vi "Get Refs of GUI Objects inside SomeTemplatesFound Tab.vi"(1 "GUI Objects":T1) -> (0 "Refs of GUI Objects inside SomeTemplatesFound Tab":refnum<vi>[](array[refnum]))   [LabVIEW 2022 SP3]
doc: "Outputs an array of Control references"
uses:
  GUI Objects (cluster).ctl
panel:
  # "Development\ncontrols/indicators useful for development and testing, but which are not outputs of the VI"
  # "Input\nInputs to the VI"
  # "Output\nOutputs of the VI"
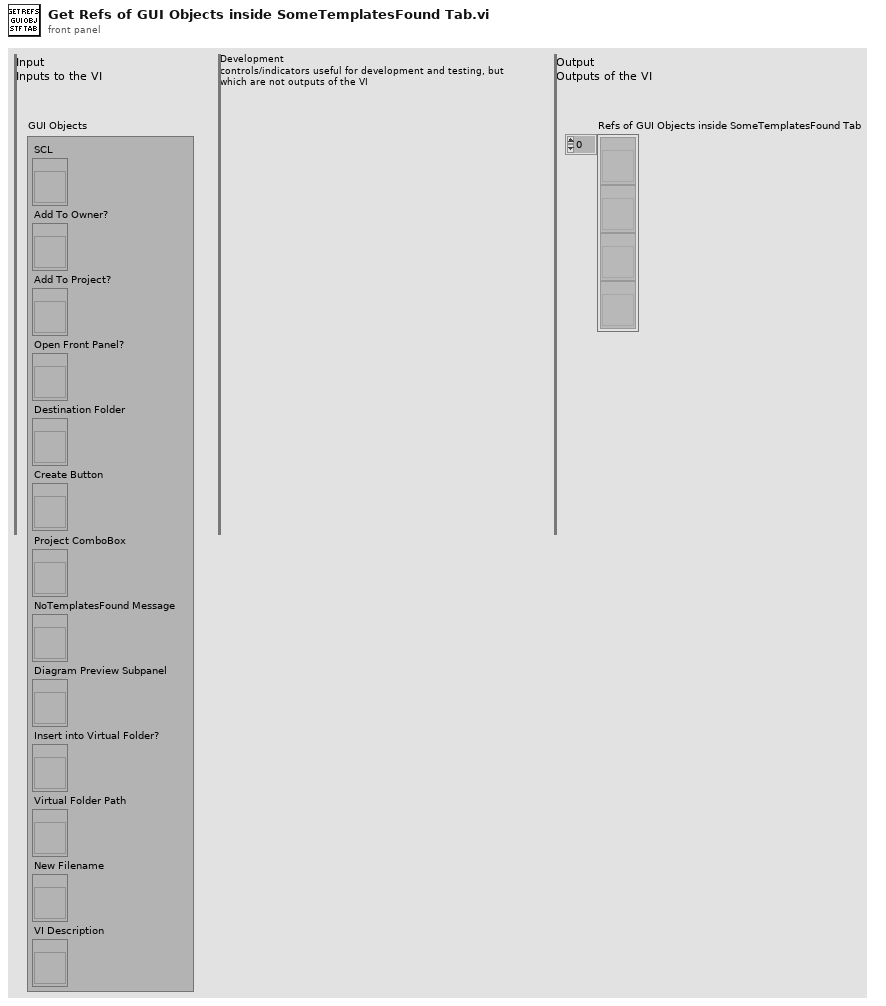
[diagram p1: front panel]
types:
  T1 = typedef "GUI Objects (cluster).ctl" = cluster{"SCL":refnum<vi>, "Add To Owner?":refnum<vi>, "Add To Project?":refnum<vi>, "Open Front Panel?":refnum<vi>, "Destination Folder":refnum<vi>, "Create Button":refnum<vi>, "Project ComboBox":refnum<vi>, "NoTemplatesFound Message":refnum<vi>, "Diagram Preview Subpanel":refnum<vi>, "Insert into Virtual Folder?":refnum<vi>, "Virtual Folder Path":refnum<vi>, "New Filename":refnum<vi>, "VI Description":refnum<vi>}
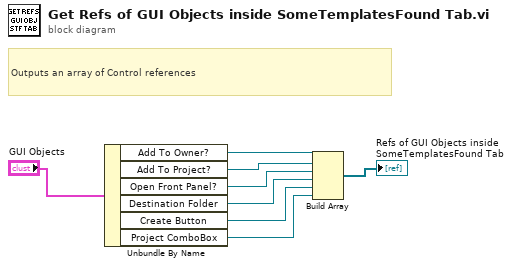
[diagram p0: block diagram]
diagram:
  # "Outputs an array of Control references"
  n1 = Unbundle By Name("GUI Objects") -> ("Add To Owner?"=w7:refnum<vi>, "Add To Project?"=w6:refnum<vi>, "Open Front Panel?"=w5:refnum<vi>, "Destination Folder"=w4:refnum<vi>, "Create Button"=w3:refnum<vi>, "Project ComboBox"=w2:refnum<vi>)
  n2 = Build Array(w7, w6, w5, w4, w3, w2) -> (→"Refs of GUI Objects inside SomeTemplatesFound Tab":refnum<vi>[])
